vi "Finish Stream.vi"(8 "error in (no error)":errorcluster, 10 "Save partial?":bool=TRUE, 11 "Photometrics Camera in":refnum<class "Photometrics Camera.lvclass">) -> (0 "error out":errorcluster, 3 "Photometrics Camera out":refnum<class "Photometrics Camera.lvclass">)   [LabVIEW 2023, in "Photometrics Camera.lvlib" / "Photometrics Camera.lvclass"]
uses:
  Photometrics Camera.lvclass
  Resources/Type Defs/Camera Type.ctl
  Photometrics Camera.lvclass/Photometrics Camera.ctl
  dcfd5c06-c9c4-48ba-9e8b-50ba9381d4b4.vi
  Camera/Camera.lvclass
  <userlib>/TPM LabVIEW adapter/Camera/Camera.lvclass
  Photometrics Camera.lvlib
panel:
  out "Dropped Frames":u64[](array[numeric])
  out "Failed?":bool[](array[boolean])
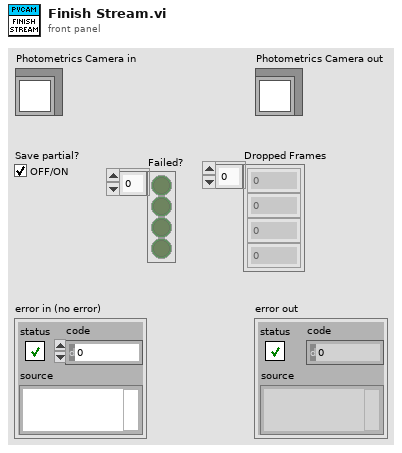
[diagram p1: front panel]
types:
  T1 = typedef "Camera Type.ctl" = enum16{"Hamamatsu", "Andor", "Photometrics"}
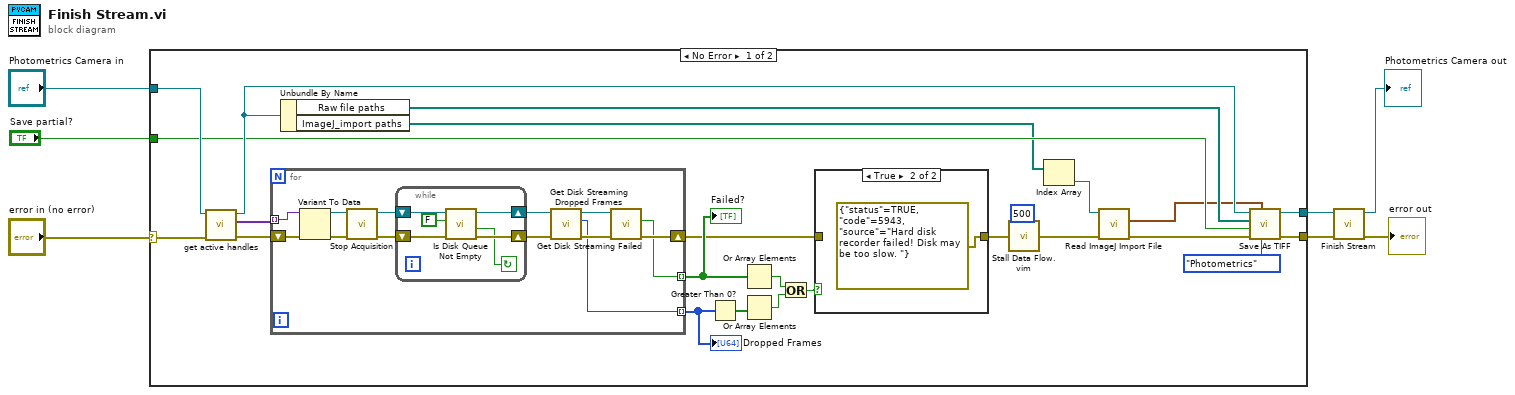
[diagram p0: block diagram]
diagram:
  n1 = case shown="No Error" "error in (no error)" {
    selector: "error in (no error)" -> [w28 w54]
    tunnel: [w25 w54] -> w4
    tunnel: "Photometrics Camera in" -> [w29 w53]
    tunnel: [w26 w53] -> w2
    tunnel: "Save partial?" -> [w14 _]
    frame No Error {
      n2 = call-dynamic "get active handles.vi"("error in (no error)"=w28, "Camera in"=w29) -> ("error out"=w31:errorcluster, "Handles"=w30:variant[], "Camera out"=w23:refnum<class "Photometrics Camera.lvclass">)  [unwired: 5 in, 2 out]
      n3 = for {
        tunnel: w30 -> [w45] mode=indexing
        shift-right: [w36] -> w16
        shift-left: w31 -> [w46]
        tunnel: [w35] -> w22 mode=indexing
        tunnel: [w34] -> w20 mode=indexing
        n4 = Variant To Data(error in=w46, Variant=w45) -> (data=w43:refnum<class "Camera.lvclass">, error out=w44:errorcluster)  [unwired: 1 in]
        n5 = call <userlib>:"Stop Acquisition.vi"("error in (no error)"=w44, "Camera in"=w43) -> ("error out"=w42:errorcluster, "Camera out"=w41:refnum<class "Camera.lvclass">)  [unwired: 8 in]
        n6 = while {
          shift-right: [w50] -> w39
          shift-left: w42 -> [w52]
          shift-right: [w48] -> w40
          shift-left: w41 -> [w51]
          stop <- w49 continue-if-true
          n7 = call <userlib>:"Is Disk Queue Not Empty.vi"("error in (no error)"=w52, "Abort Flushing To Disk"=FALSE, "Camera in"=w51) -> ("error out"=w50:errorcluster, "Disk Queue Not Empty"=w49:bool, "Camera out"=w48:refnum<class "Camera.lvclass">)  [unwired: 5 in, 1 out]
        }
        n8 = call <userlib>:"Get Disk Streaming Dropped Frames.vi"("error in (no error)"=w39, "Camera in"=w40) -> ("error out"=w38:errorcluster, "Disk Streaming Dropped Frames"=w35:u64, "Camera out"=w37:refnum<class "Camera.lvclass">)  [unwired: 7 in]
        n9 = call <userlib>:"Get Disk Streaming Failed.vi"("error in (no error)"=w38, "Camera in"=w37) -> ("error out"=w36:errorcluster, "Disk Streaming Failed"=w34:bool)  [unwired: 7 in, 1 out]
      }
      "Failed?" <- w20
      "Dropped Frames" <- w22
      n10 = Unbundle By Name(w23) -> ("Raw file paths"=w11:path[], "ImageJ_import paths"=w8:path[])
      n11 = Greater Than 0?(x=w22) -> (x > 0?=w21:bool[])
      n12 = Or Array Elements(Boolean array=w20) -> (logical OR=w18:bool)
      n13 = Or Array Elements(Boolean array=w21) -> (logical OR=w19:bool)
      n14 = Or(x=w18, y=w19) -> (x .or. y?=w17:bool)
      n15 = case shown="True" w17 {
        tunnel: w16 -> [w32 _]
        tunnel: [w32 errorcluster {"status"=TRUE, "code"=5943, "source"="Hard disk recorder failed! Disk may be too slow. "} ("error constant")] -> w15
        frame False {
        }
        frame True {
        }
      }
      n16 = call "Stall Data Flow.vim"("value in"=w15, "milliseconds to wait"=u32 500) -> ("value out"=w13:errorcluster)  [unwired: 1 out]
      n17 = Index Array(array=w8) -> (element=w10:path)  [unwired: 1 in]
      n18 = call "Read ImageJ Import File.vi"("error in"=w13, "Path In"=w10) -> ("error IO"=w12:errorcluster, "Raw File Params"=w9:cluster{"raw offset":u32, "raw frame gap":u32})  [unwired: 7 in, 1 out]
      n19 = call-dynamic "Save As TIFF.vi"("Camera Type"=Camera_Type."Photometrics", "Raw File Params"=w9, "error in (no error)"=w12, "Save partial?"=w14, "Raw file paths"=w11, "Camera in"=w23) -> ("error out"=w25:errorcluster, "Camera out"=w26:refnum<class "Photometrics Camera.lvclass">)  [unwired: 4 in]
    }
    frame Error {
    }
  }
  n20 = call-parent "Finish Stream.vi"("error in (no error)"=w4, "Camera in"=w2) -> ("error out"=→"error out":errorcluster, "Camera out"=→"Photometrics Camera out":refnum<class "Photometrics Camera.lvclass">)  [unwired: 8 in]
